vi "Call Unparameterized VI Asynchronously.vi"(0 "VI Reference":refnum<vi>) -> ()   [LabVIEW 2013]
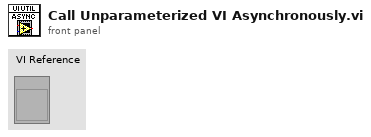
[diagram p1: front panel]
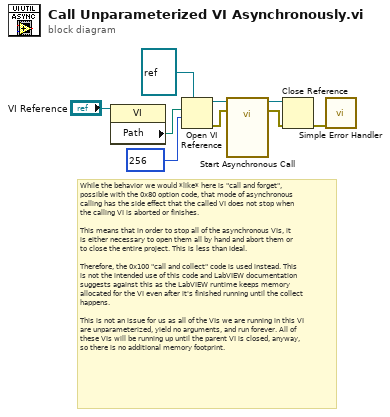
[diagram p0: block diagram]
diagram:
  # "While the behavior we would *like* here is \"call and forget\",\npossible with the 0x80 option code, that mode of asynchronous\ncalling has the side effect that the called VI does not stop when\nthe calling VI is aborted or finishes.\n\nThis means that in order to stop all of the asynchronous VIs, it\nis either necessary to open them all by hand and abort them or\nto close the entire project. This is less than ideal.\n\nTherefore, the 0x100 \"call and collect\" code is used instead. This\nis not the intended use of this code and LabVIEW documentation\nsuggests against this as the LabVIEW runtime keeps memory\nallocated for the VI even after it's finished running until the collect\nhappens. \n\nThis is not an issue for us as all of the VIs we are running in this VI\nare unparameterized, yield no arguments, and run forever. All of\nthese VIs will be running up until the parent VI is closed, anyway,\nso there is no additional memory footprint."
  n1 = property class="VI"(reference="VI Reference") -> ("Path"=w3:path)  [unwired: 1 in, 2 out]
  n2 = Open VI Reference(type specifier VI Refnum (for type only)=refnum<vi> refnum, vi path=w3, options=256) -> (vi reference=w4:refnum<vi>, error out=w5:errorcluster)  [unwired: 3 in]
  n3 = call-by-ref "Start Asynchronous Call"(reference=w4, error in=w5) -> (reference out=w6:refnum<vi>, error out=w7:errorcluster)  [unwired: 1 in]
  n4 = Close Reference(reference=w6, error in (no error)=w7) -> (error out=w8:errorcluster)
  n5 = call <vilib>:"Simple Error Handler.vi"("error in (no error)"=w8) -> ()  [unwired: 4 in, 5 out]
